vi "3D Robot Model.vi"(8 "error in (no error)":errorcluster) -> (0 "error out":errorcluster, 2 "axles":refnum<vi>[](array[refnum]), 3 "robot frame":refnum<vi>)   [LabVIEW 2015]
doc: "Creates the 3D mecanum robot object."
uses:
  <vilib>/robotics/Steering/Utilities/3D Picture/Omni Wheel Dimensions.ctl
  <vilib>/robotics/Steering/Utilities/3D Picture/Omni Wheel Colors.ctl
  <vilib>/picture/3D Picture Control/NI_3D Picture Control.lvlib
  <vilib>/robotics/Steering/Utilities/3D Picture/NI_Robotics 3D Picture Steering Utilities.lvlib
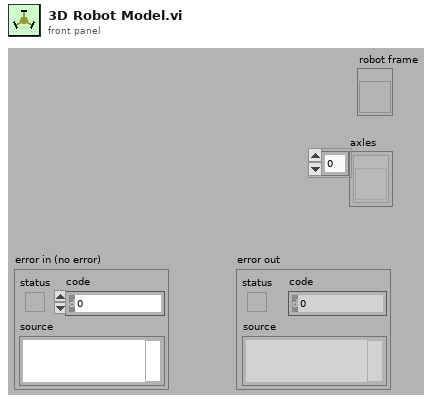
[diagram p1: front panel]
types:
  T1 = typedef "NI_Robotics 3D Picture Steering Utilities.lvlib/Omni Wheel Dimensions.ctl" = cluster{"roller thickness":dbl, "roller radius":dbl, "frame thickness":dbl, "number of rollers":i32, "axle radius":dbl, "axle length":dbl}
  T2 = typedef "NI_Robotics 3D Picture Steering Utilities.lvlib/Omni Wheel Colors.ctl" = cluster{"wheel color":u32, "roller color":u32}
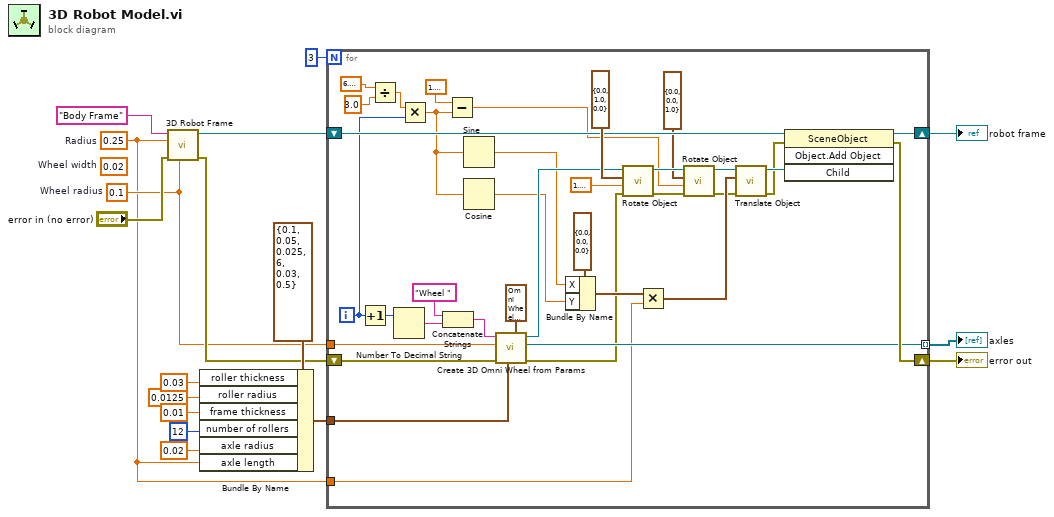
[diagram p0: block diagram]
diagram:
  w2 = 0.25  # Radius
  (unwired) 0.02  # Wheel width
  w4 = 0.1  # Wheel radius
  n1 = call "3D Robot Frame.vi"("wheel radius"=w4, "error in (no error)"="error in (no error)", "radius"=w2, "name"="Body Frame" ("Name")) -> ("error out"=w6:errorcluster, "robot frame"=w15:refnum<vi>)  [unwired: 6 in]
  n2 = Bundle By Name(cluster=T1 {"roller thickness"=0.1, "roller radius"=0.05, "frame thickness"=0.025, "number of rollers"=6, "axle radius"=0.03, "axle length"=0.5} ("drawing parameters"), "roller thickness"=0.03, "roller radius"=0.0125, "frame thickness"=0.01, "number of rollers"=12, "axle radius"=0.02, "axle length"=w2) -> (w8:T1)
  n3 = for {
    N: 3 -> [_]
    shift-right: [w48] -> w17
    shift-left: w15 -> [w46]
    tunnel: w4 -> [w43]
    tunnel: [w37] -> w16 mode=indexing
    tunnel: w8 -> [w42]
    shift-right: [w40] -> w7
    shift-left: w6 -> [w39]
    tunnel: w2 -> [w19]
    i -> [w30]
    n4 = Increment(x=w30) -> (x+1=w53:i32)
    n5 = Divide(x=6.283185307179586, y=3.0) -> (x/y=w33:dbl)
    n6 = Number To Decimal String(number=w53) -> (decimal integer string=w44:string)  [unwired: 1 out]
    n7 = Multiply(x=w33, y=w30) -> (x*y=w22:dbl)
    n8 = Concatenate Strings("Wheel " ("Name"), w44) -> (w38:string)
    n9 = Subtract(x=1.5707963267948966, y=w22) -> (x-y=w23:dbl)
    n10 = Sine(x=w22) -> (sin(x)=w21:dbl)
    n11 = Cosine(x=w22) -> (cos(x)=w20:dbl)
    n12 = call <vilib>:"Create 3D Omni Wheel from Params.vi"("colors"=T2 {"wheel color"=10449664, "roller color"=6745856}, "dimensions"=w42, "error in (no error)"=w39, "wheel radius"=w43, "name"=w38) -> ("error out"=w35:errorcluster, "rotation axis"=w37:refnum<vi>, "3D omni wheel frame"=w36:refnum<vi>)  [unwired: 4 in]
    n13 = Bundle By Name(cluster=cluster{"X":sgl, "Y":sgl, "Z":sgl} {"X"=0.0, "Y"=0.0, "Z"=0.0} ("Translation"), "X"=w21, "Y"=w20) -> (w49:cluster{"X":sgl, "Y":sgl, "Z":sgl})
    n14 = call <vilib>:"Rotate Object.vi"("error in (no error)"=w35, "Angle"=1.5707963267948966, "Axis"=cluster{"X":sgl, "Y":sgl, "Z":sgl} {"X"=0.0, "Y"=1.0, "Z"=0.0} ("Translation"), "Scene.Object In"=w36) -> ("error out"=w28:errorcluster, "Scene.Object Out"=w26:refnum<vi>)  [unwired: 6 out]
    n15 = Multiply(x=w49, y=w19) -> (x*y=w45:cluster{"X":dbl, "Y":dbl, "Z":dbl})
    n16 = call <vilib>:"Rotate Object.vi"("error in (no error)"=w28, "Angle"=w23, "Axis"=cluster{"X":sgl, "Y":sgl, "Z":sgl} {"X"=0.0, "Y"=0.0, "Z"=1.0} ("Translation"), "Scene.Object In"=w26) -> ("error out"=w27:errorcluster, "Scene.Object Out"=w25:refnum<vi>)  [unwired: 6 out]
    n17 = call <vilib>:"Translate Object.vi"("error in (no error)"=w27, "Translation"=w45, "Scene.Object In"=w25) -> ("error out"=w41:errorcluster, "Scene.Object Out"=w47:refnum<vi>)  [unwired: 7 out]
    n18 = invoke class="SceneObject" method="Object.Add Object"(reference=w46, error in=w41, "Child"=w47) -> (reference out=w48:refnum<vi>, error out=w40:errorcluster)  [unwired: 1 in, 2 out]
  }
  "robot frame" <- w17
  "axles" <- w16
  "error out" <- w7
